vi "RUSHTurret.vi"(0 "Case":dbl, 1 "Home Position":dbl, 2 "Volt Prior Home":dbl, 5 "POT":dbl, 7 "Raw Turret":dbl, 9 "Left Limit":dbl, 11 "Right Limit":dbl) -> (4 "New Case":dbl, 6 "Volt prior home":dbl, 15 "Output":dbl)   [LabVIEW 2011]
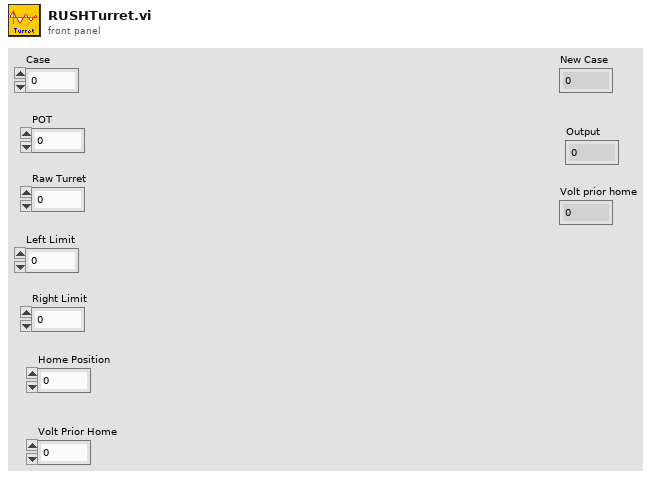
[diagram p1: front panel]
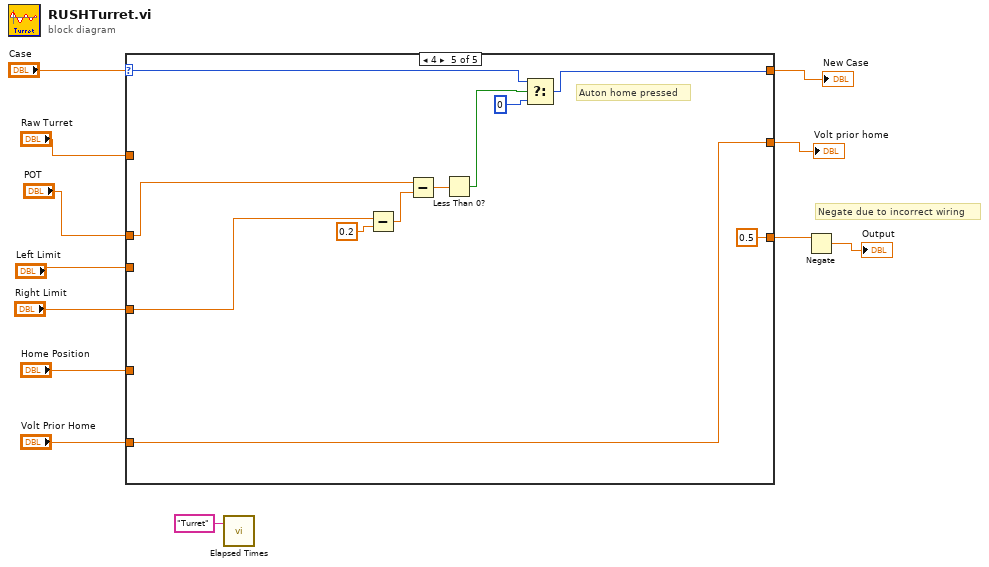
[diagram p0: block diagram]
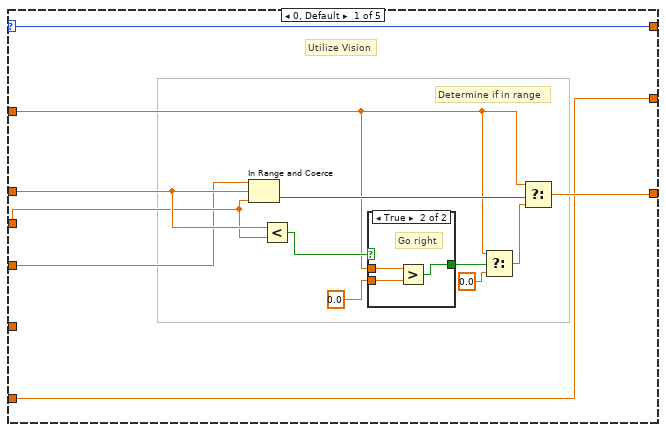
[diagram p2: hidden frame]
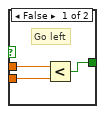
[diagram p3: hidden frame]
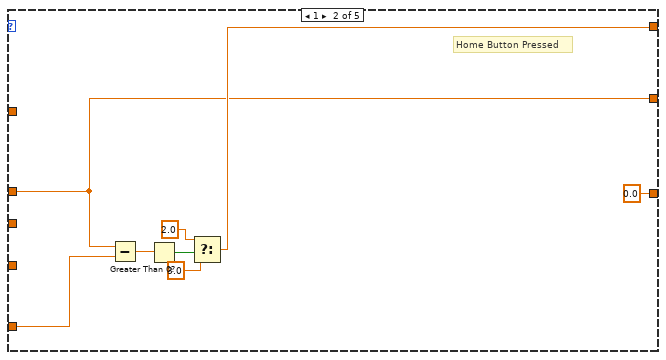
[diagram p4: hidden frame]
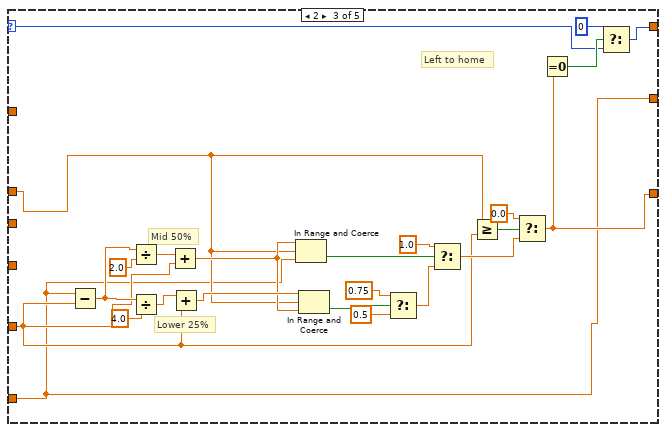
[diagram p5: hidden frame]
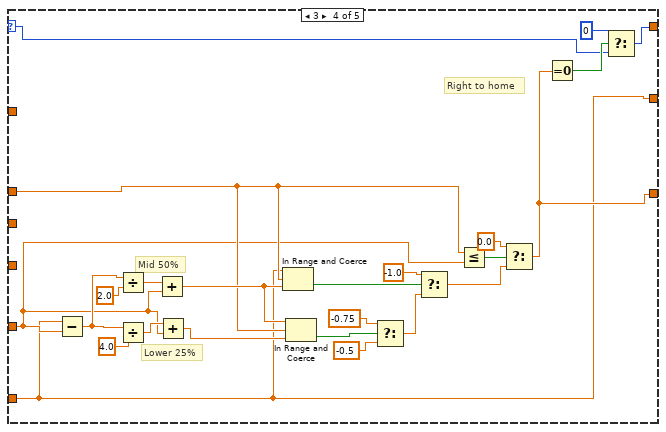
[diagram p6: hidden frame]
diagram:
  # "Negate due to incorrect wiring"
  n1 = case shown="4" "Case" {
    selector: "Case" -> [w14 _ w42 w84 w91]
    tunnel: "Raw Turret" -> [w19 _ _ _ _]
    tunnel: "POT" -> [w18 w33 w47 w67 w89]
    tunnel: "Left Limit" -> [w17 _ _ _ _]
    tunnel: "Right Limit" -> [w16 _ _ _ w88]
    tunnel: [w15 0.0 ("f") w45 w65 0.5 ("f")] -> w7
    tunnel: [w14 w34 w41 w85 w90] -> w5
    tunnel: "Home Position" -> [_ w39 w46 w66 _]
    tunnel: "Volt Prior Home" -> [w13 _ w40 w64 w98]
    tunnel: [w13 w33 w40 w64 w98] -> w2
    frame 0, Default {
      # "Determine if in range"
      # "Utilize Vision"
      n2 = In Range and Coerce(upper limit=w16, x=w18, lower limit=w17) -> (In Range?=w21:bool)  [unwired: 1 out]
      n3 = Less?(x=w18, y=w17) -> (x < y?=w20:bool)
      n4 = case shown="True" w20 {
        tunnel: 0.0 -> [w27 w31]
        tunnel: [w26 w30] -> w23
        tunnel: w19 -> [w28 w29]
        frame False {
          # "Go left"
          n5 = Less?(x=w28, y=w27) -> (x < y?=w26:bool)
        }
        frame True {
          # "Go right"
          n6 = Greater?(x=w29, y=w31) -> (0:w30:bool)
        }
      }
      n7 = Select(t=w19, s=w23, f=0.0) -> (s? t:f=w22:dbl)
      n8 = Select(t=w19, s=w21, f=w22) -> (s? t:f=w15:dbl)
    }
    frame 1 {
      # "Home Button Pressed"
      n9 = Subtract(x=w33, y=w39) -> (x-y=w38:dbl)
      n10 = Greater Than 0?(x=w38) -> (x > 0?=w37:bool)
      n11 = Select(t=2.0, s=w37, f=3.0) -> (s? t:f=w34:dbl)
    }
    frame 2 {
      # "Mid 50%"
      # "Lower 25%"
      # "Left to home"
      n12 = Subtract(x=w40, y=w46) -> (x-y=w59:dbl)
      n13 = Divide(x=w59, y=2.0) -> (x/y=w58:dbl)
      n14 = Divide(x=w59, y=4.0) -> (x/y=w57:dbl)
      n15 = Add(x=w58, y=w46) -> (x+y=w53:dbl)
      n16 = Add(x=w57, y=w46) -> (x+y=w54:dbl)
      n17 = In Range and Coerce(upper limit=w53, x=w47, lower limit=w40) -> (In Range?=w56:bool)  [unwired: 1 out]
      n18 = In Range and Coerce(upper limit=w54, x=w47, lower limit=w53) -> (In Range?=w52:bool)  [unwired: 1 out]
      n19 = Select(t=0.75, s=w52, f=0.5) -> (s? t:f=w51:dbl)
      n20 = Select(t=1.0, s=w56, f=w51) -> (s? t:f=w48:dbl)
      n21 = Greater Or Equal?(x=w47, y=w46) -> (x >= y?=w63:bool)
      n22 = Select(t=0.0, s=w63, f=w48) -> (s? t:f=w45:dbl)
      n23 = Equal To 0?(x=w45) -> (x = 0?=w44:bool)
      n24 = Select(t=0, s=w44, f=w42) -> (s? t:f=w41:i32)
    }
    frame 3 {
      # "Mid 50%"
      # "Lower 25%"
      # "Right to home"
      n25 = Subtract(x=w64, y=w66) -> (x-y=w72:dbl)
      n26 = Divide(x=w72, y=2.0) -> (x/y=w73:dbl)
      n27 = Divide(x=w72, y=4.0) -> (x/y=w74:dbl)
      n28 = Add(x=w73, y=w66) -> (x+y=w82:dbl)
      n29 = Add(x=w74, y=w66) -> (x+y=w83:dbl)
      n30 = In Range and Coerce(upper limit=w64, x=w67, lower limit=w82) -> (In Range?=w75:bool)  [unwired: 1 out]
      n31 = In Range and Coerce(upper limit=w82, x=w67, lower limit=w83) -> (In Range?=w77:bool)  [unwired: 1 out]
      n32 = Select(t=-0.75, s=w77, f=-0.5) -> (s? t:f=w78:dbl)
      n33 = Select(t=-1.0, s=w75, f=w78) -> (s? t:f=w81:dbl)
      n34 = Less Or Equal?(x=w67, y=w66) -> (x <= y?=w68:bool)
      n35 = Select(t=0.0, s=w68, f=w81) -> (s? t:f=w65:dbl)
      n36 = Equal To 0?(x=w65) -> (x = 0?=w87:bool)
      n37 = Select(t=0, s=w87, f=w84) -> (s? t:f=w85:i32)
    }
    frame 4 {
      # "Auton home pressed"
      n38 = Subtract(x=w88, y=0.2) -> (x-y=w92:dbl)
      n39 = Subtract(x=w89, y=w92) -> (x-y=w96:dbl)
      n40 = Less Than 0?(x=w96) -> (x < 0?=w95:bool)
      n41 = Select(t=w91, s=w95, f=0) -> (s? t:f=w90:i32)
    }
  }
  "New Case" <- w5
  "Volt prior home" <- w2
  n42 = call "Elapsed Times.vi"("Call Name"="Turret") -> ()  [unwired: 2 in, 1 out]
  n43 = Negate(x=w7) -> (-x=→"Output":dbl)
